vi "Unstylized UI - Run to Apply LSS Example.vi"() -> ()   [LabVIEW 2019, in "LSS.lvlib"]
doc: "This example demonstrates the application of LSS properties to a wide variety of front panel controls. The \"UI With No Styles.vi\" is what the VI looks like before application of styles, and the \"UI With No Styles - Modified.vi\" shows what the application looks like after the application of a single style sheet with many definitions.\n\nFollow instructions on the block diagram to apply styles."
uses:
  LSS.lvlib
panel:
  in  "Stop":bool
  in  "Enum":enum16{"Test", "Test2"}(ring)
  in  "Color Box":u32(colorbox)
  in  "Knob":dbl(knob) scale=0.0..10.0
  in  "Array":dbl[][](array[numeric])
  in  "Tab Control":enum32{"Page 1", "Page 2"}(tab)
  in  "OK Button":bool
  in  "Boolean 3":bool
  in  "Radio Buttons":enum32{"Radio Selection 1", "Radio Selection 2"}(radio)
  in  "Slide":dbl(slide) scale=0.0..10.0
  in  "Switch":bool
  out "Waveform Chart":dbl(graph)
  out "LED":bool
  in  "Num":dbl
  out "error out":errorcluster
  out "PathIndicator":path
  in  "PathControl":path
  in  "Combo Box":string(combo)
  in  "StringControl":string
  out "StringIndicator":string
  out "SquareLED":bool
  in  "Ring":u16(ring) items=["Test", "Test2"]
  # "See Instructions on Block Diagram"
  # "This is a free label"
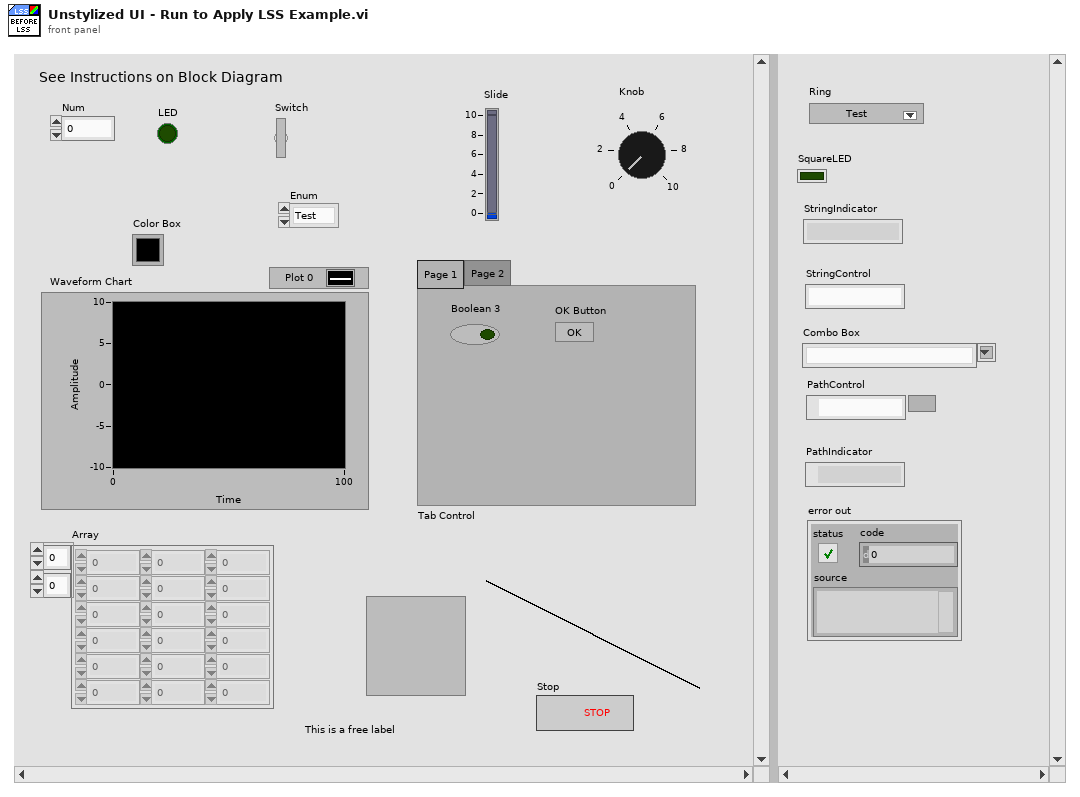
[diagram p1: front panel]
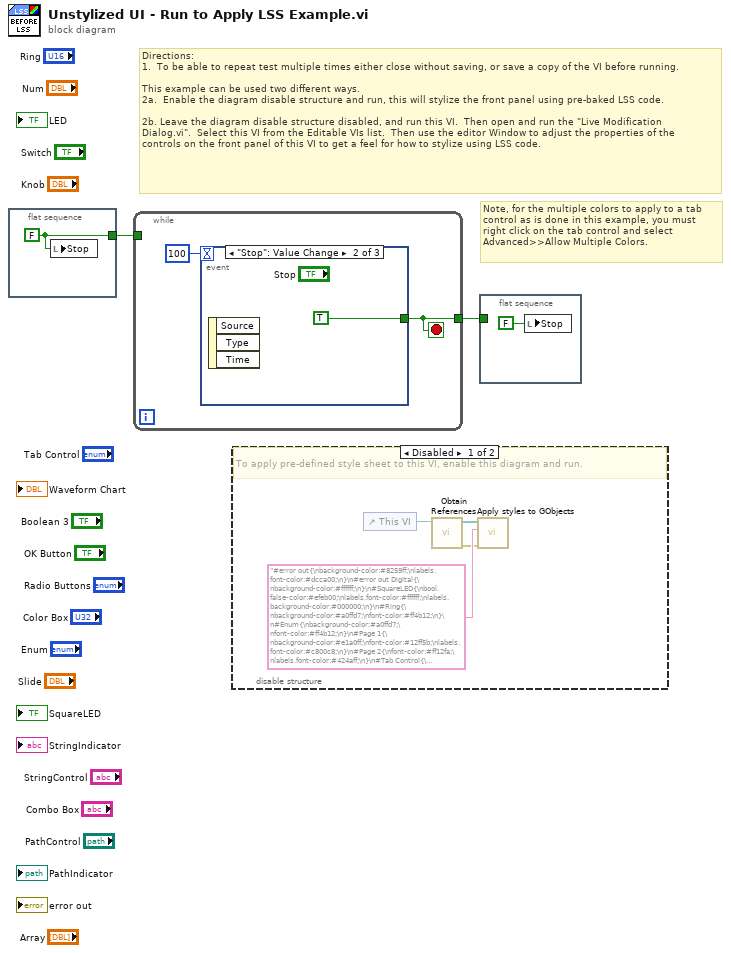
[diagram p0: block diagram]
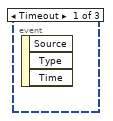
[diagram p3: hidden frame]
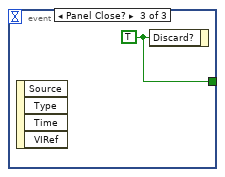
[diagram p4: hidden frame]
diagram:
  # "Note, for the multiple colors to apply to a tab\ncontrol as is done in this example, you must\nright click on the tab control and select\nAdvanced>>Allow Multiple Colors."
  # "Directions:\n1.  To be able to repeat test multiple times either close without saving, or save a copy of the VI before running.\n\nThis example can be used two different ways.\n2a.  Enable the diagram disable structure and run, this will stylize the front panel using pre-baked LSS code.\n\n2b. Leave the diagram disable structure disabled, and run this VI.  Then open and run the \"Live Modification\nDialog.vi\".  Select this VI from the Editable VIs list.  Then use the editor Window to adjust the properties of the\ncontrols on the front panel of this VI to get a feel for how to stylize using LSS code."
  n1 = flat-sequence {
    tunnel: [w3] -> w1
    frame #0 {
      w3 = FALSE ("STOP")
      n2 = local write "Stop"(w3) -> ()
    }
  }
  n3 = while {
    tunnel: [w4] -> w2
    tunnel: w1 -> [_]
    stop <- w4 stop-if-true
    n4 = event shown="[1] \"Stop\": Value Change" {
      selector: _ -> [_ _ _]
      dyn-events: _ -> [_ _ _]
      timeout: u32 100 ("milliseconds to wait") -> [_ _ _]
      tunnel: [_ TRUE w7] -> w4
      event Timeout {
        n5 = event-data() -> ()  [unwired: 1 in, 3 out]
      }
      event "Stop": Value Change {
        n6 = event-data() -> ()  [unwired: 1 in, 3 out]
      }
      event Panel Close? {
        w7 = TRUE ("Discard?")
        n7 = event-data() -> ()  [unwired: 1 in, 4 out]
        n8 = event-data("Discard?"=w7) -> ()  [unwired: 1 in, 1 out]
      }
    }
  }
  n9 = disable-structure shown="Disabled" {
    frame Disabled {
      # "To apply pre-defined style sheet to this VI, enable this diagram and run."
      n10 = control-ref of="This VI"() -> (w10:refnum<vi>)
      n11 = call "Obtain References.vi"("VI in"=w10) -> ("Error Out"=w8:errorcluster, "Front Panel Objects"=w11:refnum<vi>[])  [unwired: 9 in]
      n12 = call "Apply styles to GObjects.vi"("Error In"=w8, "Style Sheet"="#error out{\nbackground-color:#8259ff;\nlabels.font-color:#dcca00;\n}\n#error out Digital{\nbackground-color:#ffffff;\n}\n#SquareLED{\nbool.false-color:#efeb00;\nlabels.font-color:#ffffff;\nlabels.background-color:#000000;\n}\n#Ring{\nbackground-color:#a0ffd7;\nfont-color:#ff4b12;\n}\n#Enum{\nbackground-color:#a0ffd7;\nfont-color:#ff4b12;\n}\n#Page 1{\nbackground-color:#e1a0ff;\nfont-color:#12ff5b;\nlabels.font-color:#c800c8;\n}\n#Page 2{\nfont-color:#ff12fa;\nlabels.font-color:#424aff;\n}\n#Tab Control{\nbackground-color:#88caff;\n}\n#LeftPane{\nbackground-color:#b8f1ff;\nlabels.font-name:arial;\nlabels.font-size:25;\nlabels.font-color:#b009f;\n}\n#RightPane{\nbackground-color:#fefefe;\nlabels.font-name:consolas;\nlabels.font-size:25;\nlabels.font-color:#ff00df;\n}\n#Splitter{\nbackground-color:#fff388;\nlocked:true;\n}\n#Array{\nbackground-color:#000000;\n}\n#Array Digital{\nfont-color:#fff388;\n}\n#Decoration 494{\nbackground-color:#59fffd;\nfont-size:24;\nposition:300,500;\n}\n#Decoration 1004{\nbackground-color:#9f0e;\n}\n#Decoration 997{\nbackground-color:#9f0e;\n}\n#Knob{\ncolor:#fff542;\nbackground-color:#19ff00;\nfont-color:#9f0028;\n}\n#Slide{\ncolor:#fff542;\nbackground-color:#19ff00;\nfont-color:#9f0028;\n}\n#Switch{\nbool.false-color:#4cff;\nbool.true-color:#f8ff88;\n}\n#LED{\nbool.false-color:#4cff;\nbool.true-color:#f8ff88;\n}\nBoolean{\nbool.false-color:#c80048;\nbool.true-color:#bdc7e3;\n}\n#Radio Buttons{\nbackground-color:#000000;\nsize:200,120;\n}\n#Radio Selection 1{\nposition:450,265;\n}\n#Radio Selection 2{\nposition:450,320;\n}\n#Waveform Chart{\nbackground-color:#fcfcfc;\ngraph.frame-color:#cbff42;\ngraph.grid-colors.major-x:#000000;\ngraph.grid-colors.major-y:#000000;\ngraph.grid-colors.minor-x:#dcdcdc;\ngraph.grid-colors.minor-y:#dcdcdc;\nplot-color:0,#ff0000;\nfont-color:#C80028;\n}\n", "Front Panel Objects"=w11) -> ()  [unwired: 7 in, 2 out]
    }
    frame Enabled {
    }
  }
  n13 = flat-sequence {
    tunnel: w2 -> [_]
    frame #0 {
      n14 = local write "Stop"(FALSE ("STOP")) -> ()
    }
  }
